vi "Queue-Push Multiple Elements.vi"(8 "error in":errorcluster, 10 "elements":variant[](array[variant]), 11 "Buffer in":refnum<data-value>) -> (0 "error out":errorcluster, 2 "overflow":variant[](array[variant]), 3 "Buffer":refnum<data-value>)   [LabVIEW 2013, in "CircularBuffer.lvlib" / "VariantBuffer.lvclass"]
doc: "This VI allows to input an array into the buffer. The location in the buffer is updated automatically.\n\nIf the input array is larger than the buffer then just take last elements of the input array and save them in the buffer. Also give a warning that this happened."
uses:
  VariantBuffer.lvclass
  buffer-errors -- ring.ctl
  VariantBuffer.lvclass/VariantBuffer.ctl
  buffer-event -- enum.ctl
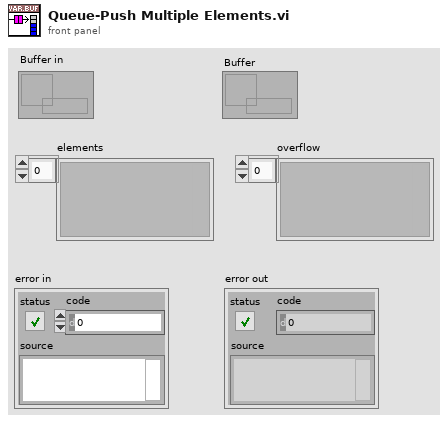
[diagram p1: front panel]
types:
  T1 = typedef "CircularBuffer.lvlib/VariantBuffer.lvclass/buffer-errors -- ring.ctl" = i32
  T2 = typedef "CircularBuffer.lvlib/VariantBuffer.lvclass/buffer-type -- enum.ctl" = enum16{"Queue", "Stack"}
  T3 = typedef "CircularBuffer.lvlib/VariantBuffer.lvclass/buffer-event -- enum.ctl" = enum16{"element-added", "element-removed", "filled", "emptied", "resized", "default-changed", "destroyed"}
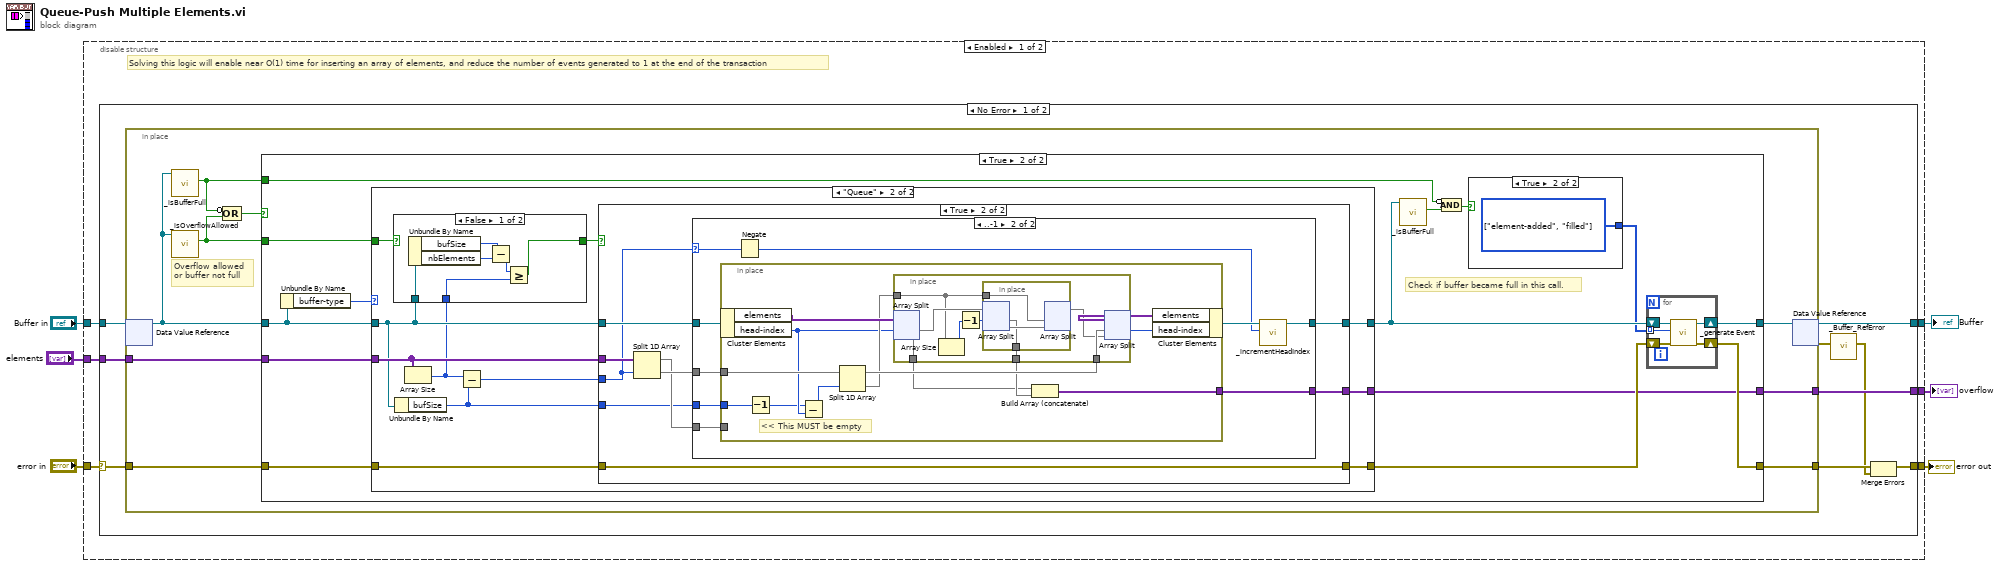
[diagram p0: block diagram]
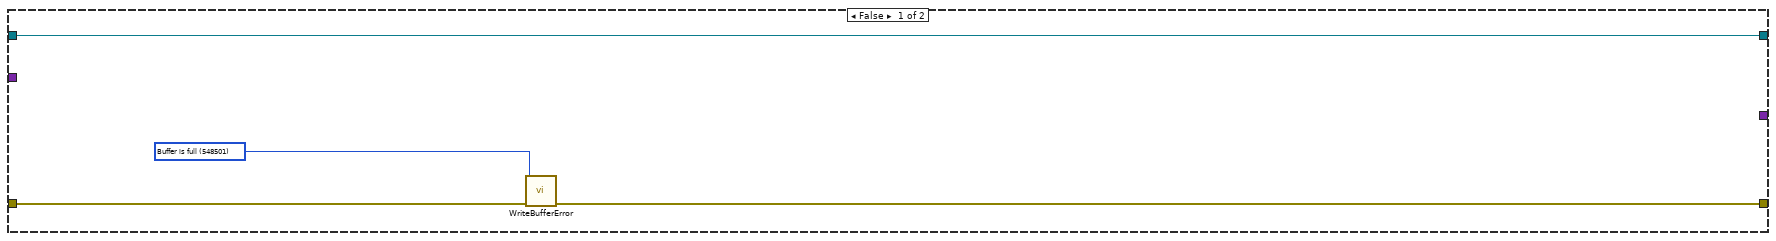
[diagram p2: hidden frame]
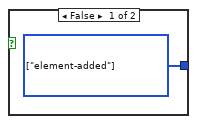
[diagram p3: hidden frame]
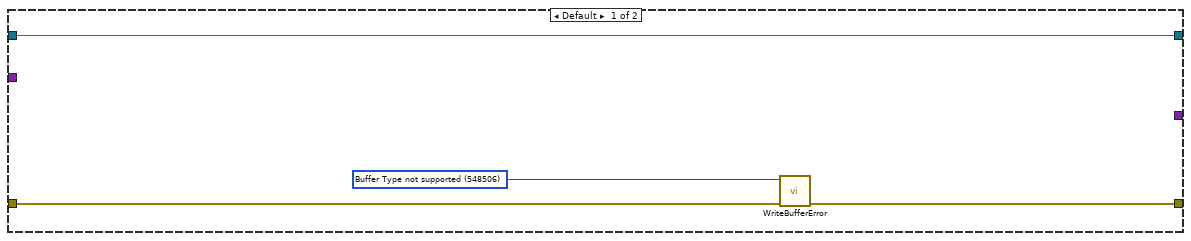
[diagram p4: hidden frame]
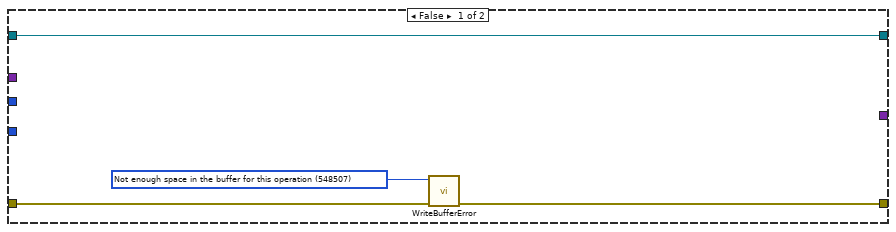
[diagram p5: hidden frame]
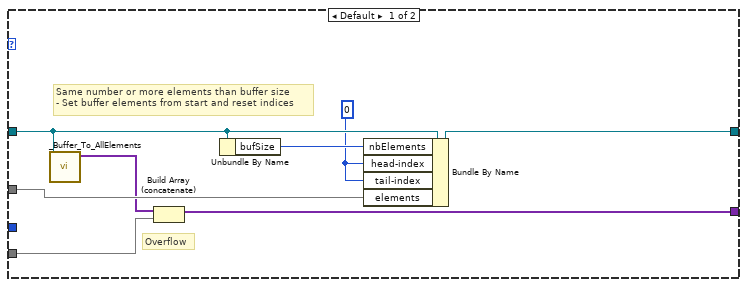
[diagram p6: hidden frame]
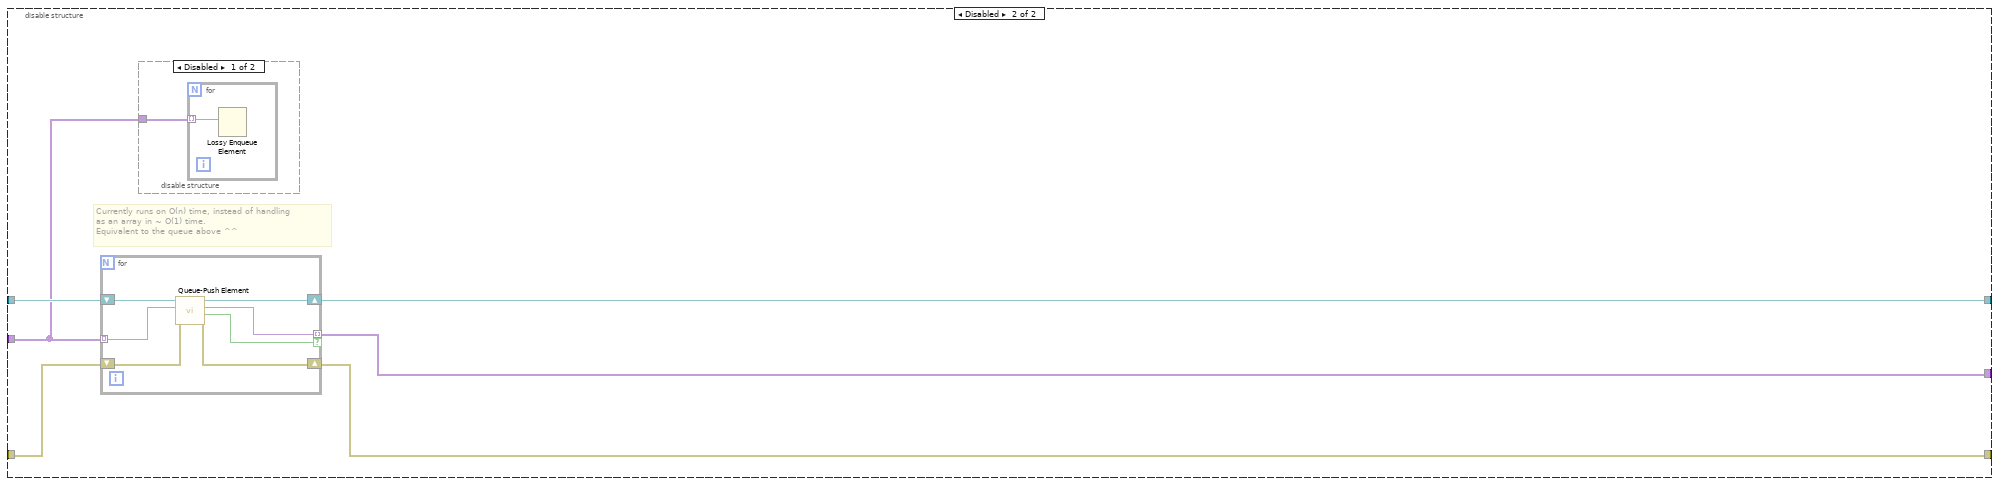
[diagram p9: hidden frame]
diagram:
  n1 = disable-structure shown="Enabled" {
    disable-tunnel: "Buffer in" -> [w12 w139]
    disable-tunnel: [w11 w138] -> w5
    disable-tunnel: [w10 w136] -> w4
    disable-tunnel: "error in" -> [w9 w137]
    disable-tunnel: "elements" -> [w8 w134]
    disable-tunnel: [w7 w135] -> w1
    frame Enabled {
      # "Solving this logic will enable near O(1) time for inserting an array of elements, and reduce the number of events generated to 1 at the end of the transaction"
      n2 = case shown="No Error" w9 {
        selector: w9 -> [w16 w133]
        tunnel: w12 -> [w21 w132]
        tunnel: [w18 w132] -> w11
        tunnel: [w20 w133] -> w10
        tunnel: w8 -> [w19 _]
        tunnel: [w17 _] -> w7
        frame No Error {
          n3 = in-place {
            in-place-border: w19 -> [w30]
            in-place-border: [w29] -> w17
            in-place-border: w16 -> [w25]
            in-place-border: [w24] -> w15
            # "Overflow allowed\nor buffer not full"
            n4 = in-place-dvr #1(w21) -> (w28:refnum<class "VariantBuffer.lvclass">)  [unwired: 1 out]
            n5 = call "_isBufferFull.vi"("VariantBuffer in"=w28) -> ("isFull"=w23:bool)  [unwired: 10 in]
            n6 = call "_isOverflowAllowed.vi"("VariantBuffer in"=w28) -> ("Allow Overflow?"=w22:bool)  [unwired: 10 in]
            n7 = Compound Arithmetic op=OR(invert w23, w22) -> (w27:bool)
            n8 = case shown="True" w27 {
              tunnel: w30 -> [_ w37]
              tunnel: [w32 w46] -> w26
              tunnel: [_ w36] -> w29
              tunnel: w28 -> [w32 w38]
              tunnel: w25 -> [w34 w47]
              tunnel: [w33 w45] -> w24
              tunnel: w23 -> [_ w39]
              tunnel: w22 -> [_ w35]
              frame False {
                w31 = T1 548501 items=["No error"=0, "Generic Buffer error"=548500, "Buffer is full"=548501, "Buffer is empty"=548502, "Buffer size cannot be 0"=548503, "Buffer reference is invalid"=548504, "Buffer event reference invalid"=548505] ("buffer-errors")
                n9 = call "WriteBufferError.vi"("error in (no error)"=w34, "buffer-errors"=w31) -> ("error out"=w33:errorcluster)  [unwired: 9 in]
              }
              frame True {
                # "Check if buffer became full in this call."
                n10 = Unbundle By Name(w38) -> ("buffer-type"=w48:T2)
                n11 = case shown="\"Queue\"" w48 {
                  tunnel: w37 -> [_ w69]
                  tunnel: [_ w68] -> w36
                  tunnel: w38 -> [w59 w62]
                  tunnel: [w59 w70] -> w43
                  tunnel: [w57 w64] -> w44
                  tunnel: w47 -> [w58 w63]
                  tunnel: w35 -> [_ w66]
                  frame Default {
                    w56 = T1 548506 items=["No error"=0, "Generic Buffer error"=548500, "Buffer is full"=548501, "Buffer is empty"=548502, "Buffer size cannot be 0"=548503, "Buffer reference is invalid"=548504, "Buffer event reference invalid"=548505, "Buffer Type not supported"=548506] ("buffer-errors")
                    n12 = call "WriteBufferError.vi"("error in (no error)"=w58, "buffer-errors"=w56) -> ("error out"=w57:errorcluster)  [unwired: 9 in]
                  }
                  frame "Queue" {
                    n13 = Unbundle By Name(w62) -> ("bufSize"=w67:i32)
                    n14 = Array Size(array=w69) -> (size(s)=w61:i32)
                    n15 = case shown="False" w66 {
                      selector: w66 -> [_ w131]
                      tunnel: [w125 w131] -> w65
                      tunnel: w62 -> [w130 _]
                      tunnel: w61 -> [w126 _]
                      frame False {
                        n16 = Unbundle By Name(w130) -> ("bufSize"=w129:i32, "nbElements"=w128:i32)
                        n17 = Subtract(x=w129, y=w128) -> (x-y=w127:i32)
                        n18 = Greater Or Equal?(x=w127, y=w126) -> (x >= y?=w125:bool)
                      }
                      frame True {
                      }
                    }
                    n19 = Subtract(x=w61, y=w67) -> (x-y=w60:i32)
                    n20 = case shown="True" w65 {
                      tunnel: [w72 w83] -> w70
                      tunnel: w69 -> [_ w82]
                      tunnel: [_ w79] -> w68
                      tunnel: w62 -> [w72 w78]
                      tunnel: w60 -> [_ w77]
                      tunnel: w67 -> [_ w76]
                      tunnel: [w73 w75] -> w64
                      tunnel: w63 -> [w74 w75]
                      frame False {
                        w71 = T1 548507 items=["No error"=0, "Generic Buffer error"=548500, "Buffer is full"=548501, "Buffer is empty"=548502, "Buffer size cannot be 0"=548503, "Buffer reference is invalid"=548504, "Buffer event reference invalid"=548505, "Buffer Type not supported"=548506, "Not enough space in the buffer for this operation"=548507] ("buffer-errors")
                        n21 = call "WriteBufferError.vi"("error in (no error)"=w74, "buffer-errors"=w71) -> ("error out"=w73:errorcluster)  [unwired: 9 in]
                      }
                      frame True {
                        n22 = Split 1D Array(array=w82, index=w77) -> (first subarray=w80:variant[], second subarray=w81:variant[])
                        n23 = case shown="..-1" w77 {
                          selector: w77 -> [_ w94]
                          tunnel: [w91 w99] -> w83
                          tunnel: w78 -> [w90 w98]
                          tunnel: w81 -> [w87 w97]
                          tunnel: w80 -> [w89 w96]
                          tunnel: [w88 w93] -> w79
                          tunnel: w76 -> [_ w95]
                          frame Default {
                            w85 = 0 ("head-index")
                            # "Overflow"
                            # "Same number or more elements than buffer size\n- Set buffer elements from start and reset indices"
                            n24 = call "_Buffer_To_AllElements.vi"("Buffer"=w90) -> ("elements"=w84:variant[])  [unwired: 10 in]
                            n25 = Build Array (concatenate)(w84, w89) -> (w88:variant[])
                            n26 = Unbundle By Name(w90) -> ("bufSize"=w86:i32)
                            n27 = Bundle By Name(cluster=w90, "nbElements"=w86, "head-index"=w85, "tail-index"=w85, "elements"=w87) -> (w91:refnum<class "VariantBuffer.lvclass">)
                          }
                          frame ..-1 {
                            n28 = in-place {
                              in-place-border: w97 -> [w103]
                              in-place-border: w96 -> [_]
                              in-place-border: w95 -> [w104]
                              in-place-border: [w108] -> w93
                              # "<< This MUST be empty"
                              n29 = in-place-cluster #2(w98) -> ("elements"=w113:variant[], "head-index"=w102:i32)
                              n30 = Decrement(x=w104) -> (x-1=w101:i32)
                              n31 = Subtract(x=w101, y=w102) -> (x-y=w110:i32)
                              n32 = Split 1D Array(array=w103, index=w110) -> (first subarray=w109:variant[], second subarray=w105:variant[])
                              n33 = in-place {
                                in-place-border: w109 -> [w121]
                                in-place-border: [w118] -> w107
                                in-place-border: [w117] -> w106
                                in-place-border: w105 -> [w116]
                                n34 = in-place-split #3(w113, w102) -> (w120:variant[], w117:variant[])
                                n35 = Array Size(array=w116) -> (size(s)=w115:i32)
                                n36 = Decrement(x=w115) -> (x-1=w114:i32)
                                n37 = in-place {
                                in-place-border: w116 -> [w124]
                                in-place-border: [w122] -> w118
                                n38 = in-place-split #4(w120, w114) -> (w122:variant[], w123:variant[])
                                n39 = in-place-split #4(w124, w123) -> (w119:variant[])  [unwired: 1 out]
                                }
                                n40 = in-place-split #3(w121, w119) -> (w112:variant[], w111:i32)
                              }
                              n41 = Build Array (concatenate)(w106, w107) -> (w108:variant[])
                              n42 = in-place-cluster #2("elements"=w112, "head-index"=w111) -> (w100:refnum<class "VariantBuffer.lvclass">)
                            }
                            n43 = Negate(x=w94) -> (-x=w92:i32)
                            n44 = call "_incrementHeadIndex.vi"("NbElements"=w92, "VariantBuffer in"=w100) -> ("VariantBuffer out"=w99:refnum<class "VariantBuffer.lvclass">)  [unwired: 9 in]
                          }
                        }
                      }
                    }
                  }
                }
                n45 = call "_isBufferFull.vi"("VariantBuffer in"=w43) -> ("isFull"=w42:bool)  [unwired: 10 in]
                n46 = Compound Arithmetic op=AND(invert w39, w42) -> (w41:bool)
                n47 = case shown="True" w41 {
                  tunnel: [w49 w50] -> w40
                  frame False {
                    w49 = T3[] [enum."element-added"] items=["element-added", "element-removed", "filled", "emptied", "resized", "default-changed", "destroyed"]
                  }
                  frame True {
                    w50 = T3[] [enum."element-added", enum."filled"] items=["element-added", "element-removed", "filled", "emptied", "resized", "default-changed", "destroyed"]
                  }
                }
                n48 = for {
                  tunnel: w40 -> [w53] mode=indexing
                  shift-right: [w55] -> w46
                  shift-left: w43 -> [w54]
                  shift-right: [w52] -> w45
                  shift-left: w44 -> [w51]
                  n49 = call "_generate Event.vi"("error in"=w51, "event"=w53, "VariantBuffer"=w54) -> ("error out"=w52:errorcluster, "VariantBuffer out"=w55:refnum<class "VariantBuffer.lvclass">)  [unwired: 7 in]
                }
              }
            }
            n50 = in-place-dvr #1(w26) -> (w18:refnum<data-value>, w14:errorcluster)
          }
          n51 = call "_Buffer_RefError.vi"("error in (no error)"=w14) -> ("error out"=w13:errorcluster)  [unwired: 10 in]
          n52 = Merge Errors(w15, w13) -> (w20:errorcluster)
        }
        frame Error {
        }
      }
    }
    frame Disabled {
      # "Currently runs on O(n) time, instead of handling\nas an array in ~ O(1) time.\nEquivalent to the queue above ^^"
      n53 = for {
        tunnel: w134 -> [w147] mode=indexing
        shift-right: [w144] -> w138
        shift-left: w139 -> [w148]
        shift-right: [w145] -> w136
        shift-left: w137 -> [w146]
        tunnel: [w143] -> w135 mode=indexing if=w142
        n54 = call "Queue-Push Element.vi"("error in"=w146, "element"=w147, "Buffer in"=w148) -> ("error out"=w145:errorcluster, "overflowed"=w142:bool, "overflow"=w143:variant, "Buffer"=w144:refnum<data-value>)  [unwired: 4 in, 1 out]
      }
      n55 = disable-structure shown="Disabled" {
        disable-tunnel: w134 -> [w140 _]
        frame Disabled {
          n56 = for {
            tunnel: w140 -> [w141] mode=indexing
            n57 = Lossy Enqueue Element(element=w141) -> ()  [unwired: 2 in, 4 out]
          }
        }
        frame Enabled {
        }
      }
    }
  }
  "error out" <- w4
  "Buffer" <- w5
  "overflow" <- w1
